vi "Interpret string.vi"(8 "error in (no error)":errorcluster, 10 "String":string, 11 "Cluster":T1={"Command"=enum."£ncal", "data"=variant}) -> (0 "error out":errorcluster, 1 "Numeric 2":dbl, 2 "Numeric":u16, 3 "String 2":string)   [LabVIEW 2016]
uses:
  Controls/Command cluster.ctl
  Controls/Command list.ctl
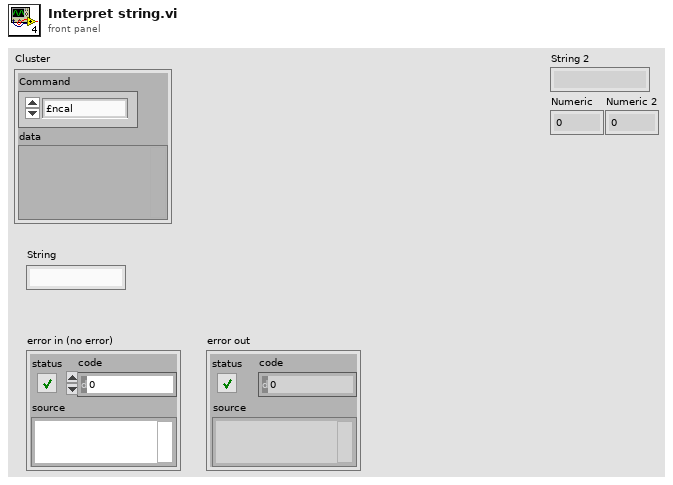
[diagram p1: front panel]
types:
  T1 = typedef "Command cluster.ctl" = cluster{"Command":T2, "data":variant}
  T2 = typedef "Command list.ctl" = enum16{"", "£nabort", "getaxisno", "£getserialno", "£nidentify", "&&£setnlimit", "&£nm", "&£snv", "&£speed", "£np", "£ncal"}
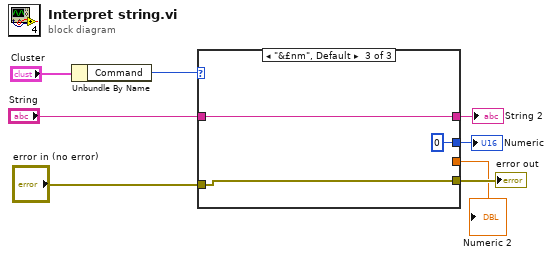
[diagram p0: block diagram]
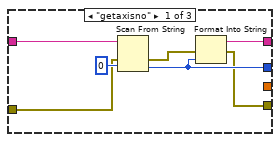
[diagram p2: hidden frame]
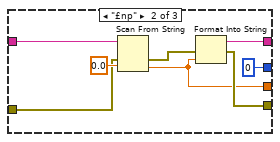
[diagram p3: hidden frame]
diagram:
  n1 = Unbundle By Name("Cluster") -> ("Command"=w7:T2)
  n2 = case shown="\"&£nm\", Default" w7 {
    tunnel: "error in (no error)" -> [w14 w22 w26]
    tunnel: [w10 w19 w26] -> w5
    tunnel: "String" -> [w13 w21 w25]
    tunnel: [w9 w18 w25] -> w3
    tunnel: [w12 u16 0 u16 0] -> w2
    tunnel: [_ w16 _] -> w1
    frame "getaxisno" {
      n3 = Scan From String(input string=w13, error in=w14, default 1=u16 0) -> (error out=w11:errorcluster, output 1=w12:u16)  [unwired: 2 in, 2 out]
      n4 = Format Into String(error in=w11, w12) -> (resulting string=w9:string, error out=w10:errorcluster)  [unwired: 2 in]
    }
    frame "£np" {
      n5 = Scan From String(input string=w21, error in=w22, default 1=0.0) -> (error out=w20:errorcluster, output 1=w16:dbl)  [unwired: 2 in, 2 out]
      n6 = Format Into String(error in=w20, w16) -> (resulting string=w18:string, error out=w19:errorcluster)  [unwired: 2 in]
    }
    frame "&£nm", Default {
    }
  }
  "error out" <- w5
  "String 2" <- w3
  "Numeric" <- w2
  "Numeric 2" <- w1
